vi "Read Supported Functions.vi"(8 "error in (no error)":errorcluster, 11 "Source in":refnum<class "Source.lvclass">) -> (0 "error out":errorcluster, 2 "Supported Functions":T1[](array[typedef]), 3 "Source out":refnum<class "Source.lvclass">)   [LabVIEW 2015, in "Source.lvclass"]
uses:
  Source.lvclass
  Mag Lab Hardware Function.ctl
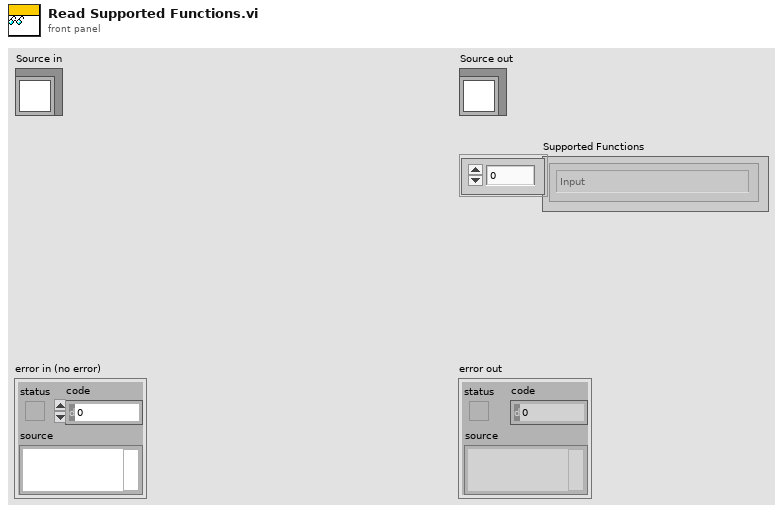
[diagram p1: front panel]
types:
  T1 = typedef "Mag Lab Hardware Function.ctl" = enum16{"Input", "Voltmeter", "Output", "Current source", "Digitizer", "Temperature controller"}
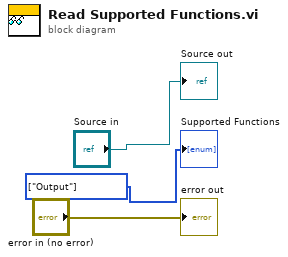
[diagram p0: block diagram]
diagram:
  w1 = T1[] [enum."Output"] items=["Input", "Voltmeter", "Output", "Current source", "Digitizer", "Temperature controller"] ("Supported Functions")
  "error out" <- "error in (no error)"
  "Source out" <- "Source in"
  "Supported Functions" <- w1
